vi "IPS Read Switch Heater NOT WORKING.vi"(4 "Error In":errorcluster={"status"=FALSE, "code"=1073676294, "source"="VISA Read in Prologix USB GPIB Command.vi"}, 6 "Target Field (T)":dbl, 7 "VISA resource name":refnum<visa-resource-name>="GPIB1::25::INSTR") -> (0 "Error Out":errorcluster={"status"=TRUE, "code"=-1073807346, "source"="VISA Open in NI USB GPIB Command.vi->IPS Set Target Field.vi->IV_B_2Gates_4461-4462.vi"}, 1 "Response":string, 3 "VISA resource name":refnum<visa-resource-name>)   [LabVIEW 2016, in "IPS-120.lvlib"]
uses:
  IPS-120.lvlib
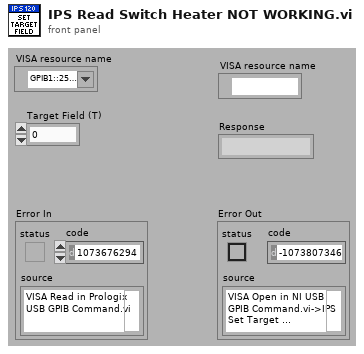
[diagram p1: front panel]
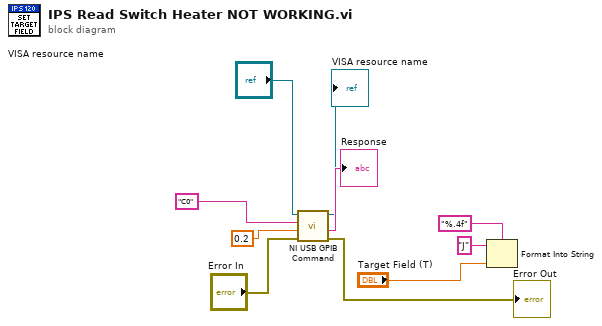
[diagram p0: block diagram]
diagram:
  n1 = call "NI USB GPIB Command.vi"("Error In"="Error In", "Wait for instrument to respond (s)"=0.2, "String to Send"="C0", "VISA resource name"="VISA resource name") -> ("Error Out"=→"Error Out":errorcluster, "Return String from Device (Not all commands return a String)"=→"Response":string, "VISA resource name out"=→"VISA resource name":refnum<visa-resource-name>)  [unwired: 1 out]
  n2 = Format Into String(format string="%.4f", initial string="J" ("string (\"\")"), "Target Field (T)") -> ()  [unwired: 1 in, 2 out]
